vi "Error.vi"(8 "error in (no error)":errorcluster, 11 "Queue in":refnum<queue>) -> (0 "error out":errorcluster)   [LabVIEW 2019, in "Prueba04.lvclass"]
uses:
  Prueba04.lvclass
  Prueba/Queues/Private Controls/Control HMI Data Cluster.ctl
  Prueba/Queues/Private Controls/Estados.ctl
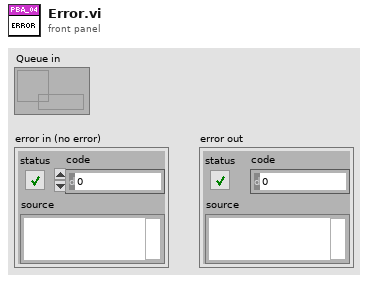
[diagram p1: front panel]
types:
  T1 = typedef "Control HMI Data Cluster.ctl" = cluster{"Estados":T2, "Data":variant}
  T2 = typedef "Estados.ctl" = enum16{"CargaReferencias", "LeerArchivoConfiguracion", "RevisaTipoGenerador", "inicio", "conf_instru", "escribe_frec", "lee_BD", "lee_referencia", "guardarVrefA", "guardarVrefC", "guardarVrefZ", "FrecAmp_A1", "FrecAmp_C1", "FrecAmp_Z1", "FrecAmp_A2", "FrecAmp_C2", "FrecAmp_Z2", "iniciarGEN", "monitoreo", "detenerGEN", "crea_voltajes_prueba_A", "crea_voltajes_prueba_C", "crea_voltajes_prueba_Z", "voltajeInicialA2", "voltajeInicialC2", "voltajeInicialZ2", "actualizarVrefA", "actualizarVrefC", "actualizarVrefZ", "ingresaMedicionesA", "ingresaMedicionesC", "ingresaMedicionesZ", "cumplimiento", "listo_evaluar", "evaluar", "final", "guardaMedicionesA", "guardaMedicionesC", "guardaMedicionesZ", "ultimaFrec", "generaA2", "detieneA2", "salir", "Error"}
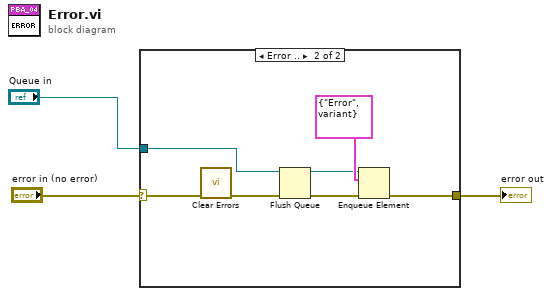
[diagram p0: block diagram]
diagram:
  n1 = case shown="Error .." "error in (no error)" {
    selector: "error in (no error)" -> [w4 w9]
    tunnel: "Queue in" -> [_ w6]
    tunnel: [w4 w11] -> w2
    frame No Error {
    }
    frame Error {
      n2 = call <vilib>:"Clear Errors.vi"("error in (no error)"=w9) -> ("error out"=w8:errorcluster)  [unwired: 5 in, 1 out]
      n3 = Flush Queue(queue=w6, error in (no error)=w8) -> (queue out=w5:refnum<queue>, error out=w7:errorcluster)  [unwired: 1 out]
      n4 = Enqueue Element(queue=w5, element=T1 {"Estados"=enum."Error", "Data"=variant}, error in (no error)=w7) -> (error out=w11:errorcluster)  [unwired: 1 in, 2 out]
    }
  }
  "error out" <- w2
